vi "DRC Send Calibration.vi"(2 "Calibration #":i32=6 min=5 max=31, 3 "Sensor Type":i32(ring) items=["Carbon Glass", "Platinum", "Diode"], 4 "GPIB Address (VISA)":refnum<visa-resource-name>) -> (0 "Curve Table for this Calibration":string, 1 "Sensor Curve Information Table":string)   [LabVIEW 2024]
doc: "This VI loads a calibration file into the Lakeshore DRC 93C or 82C temperature controller. The file is a line of up to 18 characters of ID info, followed by the temperature information in 2 columns of temperature and resistance (sensor value). The columns may be separated by any character. Lines beginning with a \"#\" are ignored. The file can be in any order and is sorted in order of increasing sensor value.\nScott Hannahs, NHMFL-FSU December 1995"
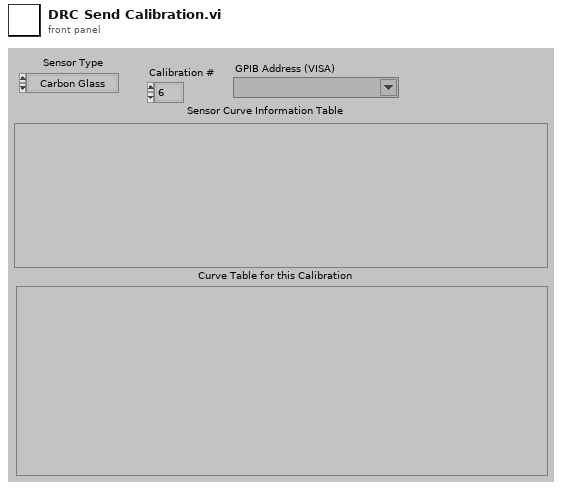
[diagram p1: front panel]
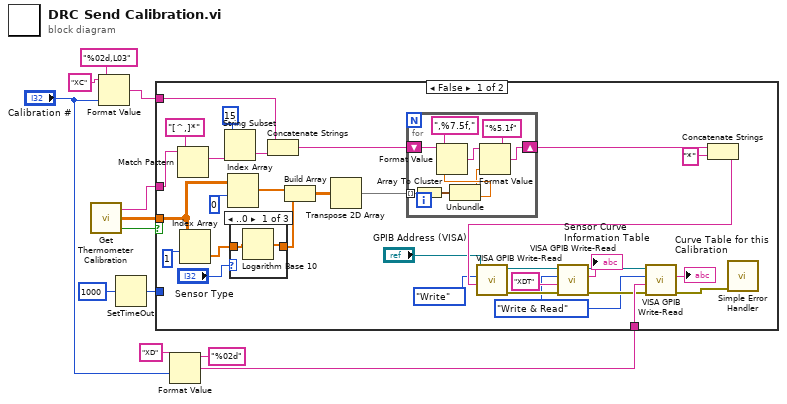
[diagram p0: block diagram]
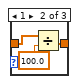
[diagram p2: hidden frame]
diagram:
  n1 = call "Get Thermometer Calibration.vi"() -> ("Cancelled"=w7:bool, "Thermometer Calibration Data"=w4:dbl[][], "ID String"=w6:string)
  n2 = Format Value(string ("")="XC", format string="%02d,L03", value (0)="Calibration #") -> (output string=w5:string)
  n3 = SetTimeOut(1:1000) -> (0:w2:i32)
  n4 = Format Value(string ("")="XD", format string="%02d", value (0)="Calibration #") -> (output string=w1:string)
  n5 = case shown="False" w7 {
    tunnel: w6 -> [w39 _]
    tunnel: w5 -> [w38 _]
    tunnel: w4 -> [w34 _]
    tunnel: w2 -> [_ _]
    tunnel: w1 -> [w24 _]
    frame False {
      w16 = enum16{"Write", "Read", "Write & Read"}."Write & Read" ("Action")
      n6 = Match Pattern(string=w39, regular expression="[^,]*") -> (match substring=w43:string)  [unwired: 1 in, 3 out]
      n7 = Index Array(array=w34, index (row)=1) -> (element=w36:dbl[])  [unwired: 1 in]
      n8 = String Subset(string=w43, length (rest)=15) -> (substring=w41:string)  [unwired: 1 in]
      n9 = Index Array(array=w34, index (row)=0) -> (element=w33:dbl[])  [unwired: 1 in]
      n10 = case shown="..0" "Sensor Type" {
        tunnel: [w54 w57 w58] -> w35
        tunnel: w36 -> [w53 w55 w58]
        frame ..0 {
          n11 = Logarithm Base 10(1:w53) -> (0:w54:dbl[])
        }
        frame 1 {
          n12 = Divide(x=w55, y=100.0) -> (x/y=w57:dbl[])
        }
        frame 2.. {
        }
      }
      n13 = Concatenate Strings(w38, w41) -> (w31:string)
      n14 = Build Array(w33, w35) -> (w32:dbl[][])
      n15 = Transpose 2D Array(2D array=w32) -> (transposed array=w18:dbl[][])
      n16 = for {
        shift-right: [w44] -> w29
        shift-left: w31 -> [w45]
        tunnel: w18 -> [w51] mode=indexing
        n17 = Array To Cluster(array=w51) -> (cluster=w52:cluster{"[0]":dbl, "[1]":dbl})
        n18 = Unbundle(w52) -> ("[0]"=w46:dbl, "[1]"=w47:dbl)
        n19 = Format Value(string ("")=w45, format string=",%7.5f,", value (0)=w47) -> (output string=w49:string)
        n20 = Format Value(string ("")=w49, format string="%5.1f", value (0)=w46) -> (output string=w44:string)
      }
      n21 = Concatenate Strings(w29, "*") -> (w28:string)
      n22 = call "VISA GPIB Write-Read.vi"("Command"=w28, "Action"=enum16{"Write", "Read", "Write & Read"}."Write", "VISA resource name"="GPIB Address (VISA)") -> ("error out"=w26:errorcluster, "dup VISA Session"=w15:refnum<visa-resource-name>)  [unwired: 5 in, 2 out]
      n23 = call "VISA GPIB Write-Read.vi"("error in (no error)"=w26, "Command"="XDT", "Action"=w16, "VISA resource name"=w15) -> ("error out"=w23:errorcluster, "String Returned"=→"Sensor Curve Information Table":string, "dup VISA Session"=w14:refnum<visa-resource-name>)  [unwired: 4 in, 1 out]
      n24 = call "VISA GPIB Write-Read.vi"("error in (no error)"=w23, "Command"=w24, "Action"=w16, "VISA resource name"=w14) -> ("error out"=w21:errorcluster, "String Returned"=→"Curve Table for this Calibration":string)  [unwired: 4 in, 2 out]
      n25 = call <vilib>:"Simple Error Handler.vi"("error in (no error)"=w21) -> ()  [unwired: 4 in, 5 out]
    }
    frame True {
    }
  }
